vi "Setup UI.vi"(8 "error in (no error)":errorcluster, 10 "Set UI to input? (F)":bool, 11 "anritsu reader in":refnum<class "anritsu reader.lvclass">) -> (0 "error out":errorcluster, 3 "anritsu reader out":refnum<class "anritsu reader.lvclass">)   [LabVIEW 2017, in "anritsu reader.lvclass"]
doc: "Setup UI constructs an object -- populates its member fields -- from a front panel the user can see. The VI should be as simple as possible so that a UI loop can poll it continuously for updates. \n\nThe VI is designed to be used as a subPanel within another VI. Wire true to \"Set UI to input\" only on the first call, just after inserting this VI into a subPanel, to populate its controls with the class's current values.\n\nSetup UI is distinct from the class constructor. Class constructors are not polymorphic, yet configure dialogs need to configure objects without knowing their type -- and polymorphism is the necessary solution. Thus, Setup UI is a polymorphic class constructor. This continously polled \"Setup UI\" concept is a kludge: a better idea would be an XControl, but those require a steeper learning curve."
uses:
  anritsu reader.lvclass
  Instruments/Anritsu Power Meter/Anritsu Power Meter/Public/Averaging control.ctl
  Instruments/Anritsu Power Meter/Anritsu Power Meter/Public/Display control.ctl
  Instruments/Anritsu Power Meter/Anritsu Power Meter/Public/Measuring rate control.ctl
  Instruments/Anritsu Power Meter/Anritsu Power Meter/Public/Range control watts and dBm.ctl
  Instruments/Anritsu Power Meter/Anritsu Power Meter/Public/Auto Range control.ctl
  anritsu reader.lvclass/anritsu reader.ctl
  Reader/Reader.lvclass
panel:
  in  "Auto Ranging?":T1
  in  "Unit Range":T2
  in  "Calibration Factor":dbl
  in  "Measuring rate":T3
  in  "Units":T4
  in  "Averaging":T5
  # "Anritsu Power Meter Control Setup"
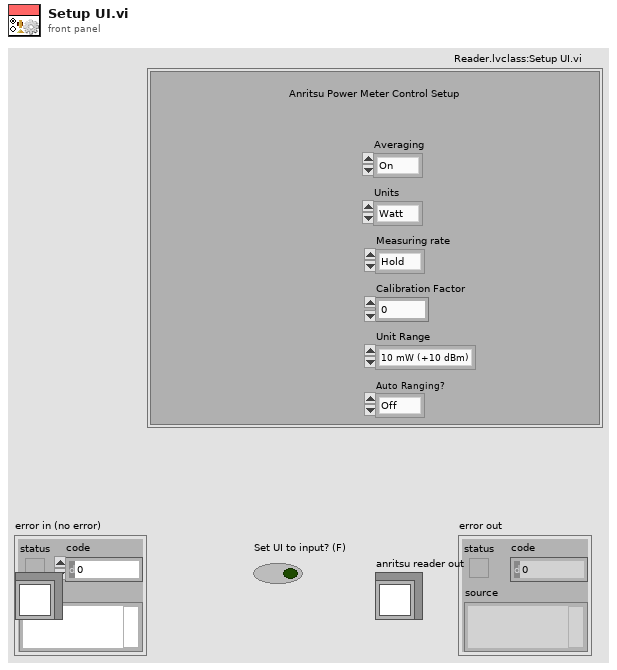
[diagram p1: front panel]
types:
  T1 = typedef "Auto Range control.ctl" = enum16{"Off", "On"}
  T2 = typedef "Range control watts and dBm.ctl" = enum16{"10 mW (+10 dBm)", "1 mW (0 dBm)", "100 uW (-10 dBm)", "10 uW (-20 dBm)", "1 uW (-30 dBm)", "100 nW (-40 dBm)", "10 nW (-50 dBm)", "1 nW (-60 dBm)", "100 pW (-70 dBm)", "10 pW (-80 dBm)"}
  T3 = typedef "Measuring rate control.ctl" = enum16{"Hold", "Free Run", "Exit Trigger"}
  T4 = typedef "Display control.ctl" = enum16{"Watt", "dBm", "dB (REL)"}
  T5 = typedef "Averaging control.ctl" = enum16{"On", "Off"}
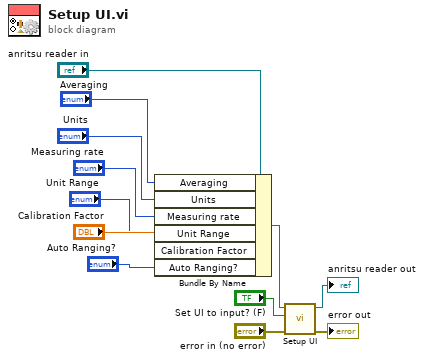
[diagram p0: block diagram]
diagram:
  n1 = Bundle By Name(cluster="anritsu reader in", "Averaging"="Averaging", "Units"="Units", "Measuring rate"="Measuring rate", "Unit Range"="Unit Range", "Calibration Factor"="Calibration Factor", "Auto Ranging?"="Auto Ranging?") -> (w7:refnum<class "anritsu reader.lvclass">)
  n2 = call-parent "Setup UI.vi"("error in (no error)"="error in (no error)", "Set UI to input? (F)"="Set UI to input? (F)", "Reader in"=w7) -> ("error out"=→"error out":errorcluster, "Reader out"=→"anritsu reader out":refnum<class "anritsu reader.lvclass">)  [unwired: 7 in]
